vi "usbdlllib.vi"   [LabVIEW 2013, in "libusvlv.lvlib"]
uses:
  libusvlv.lvlib
  UsbCom.dll
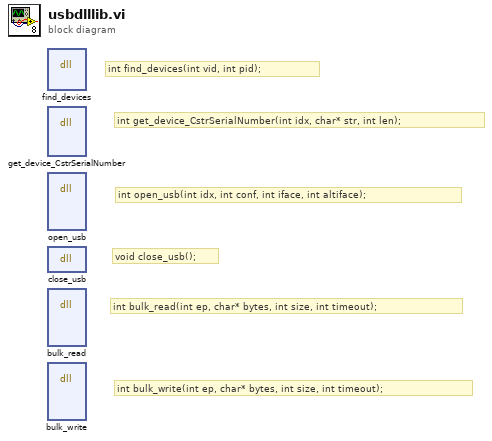
[diagram p0: block diagram]
diagram:
  # "int bulk_read(int ep, char* bytes, int size, int timeout);"
  # "int bulk_write(int ep, char* bytes, int size, int timeout);"
  # "void close_usb();"
  # "int open_usb(int idx, int conf, int iface, int altiface);"
  # "int get_device_CstrSerialNumber(int idx, char* str, int len);"
  # "int find_devices(int vid, int pid);"
  n1 = dll-call lib="E:/libusvlv/UsbCom.dll" fn="find_devices"() -> ()  [unwired: 8 in, 2 out]
  n2 = dll-call lib="E:/libusvlv/UsbCom.dll" fn="get_device_CstrSerialNumber"() -> ()  [unwired: 10 in, 2 out]
  n3 = dll-call lib="E:/libusvlv/UsbCom.dll" fn="open_usb"() -> ()  [unwired: 12 in, 2 out]
  n4 = dll-call lib="E:/libusvlv/UsbCom.dll" fn="close_usb"() -> ()  [unwired: 4 in, 2 out]
  n5 = dll-call lib="E:/libusvlv/UsbCom.dll" fn="bulk_read"() -> ()  [unwired: 12 in, 2 out]
  n6 = dll-call lib="E:/libusvlv/UsbCom.dll" fn="bulk_write"() -> ()  [unwired: 12 in, 2 out]
